vi "Wait for Win Msg.vi"(0 "win msg queue":T1, 1 "ms timeout (-1)":i32=-1, 2 "ignore previous (F)":bool, 3 "error in (no error)":errorcluster) -> (4 "Messages Remaining in Queue":i32, 5 "Sent":bool, 6 "win msg queue out":T1, 7 "Message":T2 {"Msg" format="%.0x"; "hWnd" format="%.0x"}, 8 "timed out":bool, 9 "error out":errorcluster)   [LabVIEW 2011]
doc: "Asynchronously waits for the next windows message that is added to the queue and returns it. If ignore previous is set to true, all messages occurring before this wait are deleted. If it is set to false and prior messages are waiting in the queue, this VI returns immediately with the next message. No more than one Wait per queue should be active at any given time. Simultaneous waits on different queues are permissible.\n\nParameters:\nwin msq queue: the queue for which to wait.\n\nms timeout: timeout time in milliseconds\n\niqnore previous: whether to pay attention to messages added to the queue before this VI begins waiting. If true, only the message added to the queue while the VI is waiting are detected. All other prior messages are deleted. If false, if one or more messages are posted before the VI begins waiting, this VI returns immediately with the oldest message in the queue.\n\ntimed out: returns true if the timeout expired.\n\nMessage: the oldest message in the queue is removed and returned. (Usually this is the only message in the queue.) See Get Next Message.vi for more information.\n\nSent: returns true if the returned message was sent to the window (via SendMessage) or false if it was posted (via PostMessage). Note: messages that are sent will not have valid time or point parameters.\n\nMessage Remaining: the number of messsages still in the queue.\n\nErrors:\n6751: not a valid windows message queue.\n6752: no messages in queue when read was attempted."
uses:
  Win Msg Q RefNum.ctl
  Win Msg.ctl
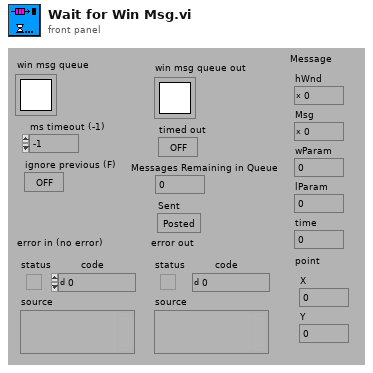
[diagram p1: front panel]
types:
  T1 = typedef "Win Msg Q RefNum.ctl" = refnum<k1>
  T2 = typedef "Win Msg.ctl" = cluster{"hWnd":u32, "Msg":u32, "wParam":u32, "lParam":i32, "time":u32, "point":cluster{"X":i32, "Y":i32}}
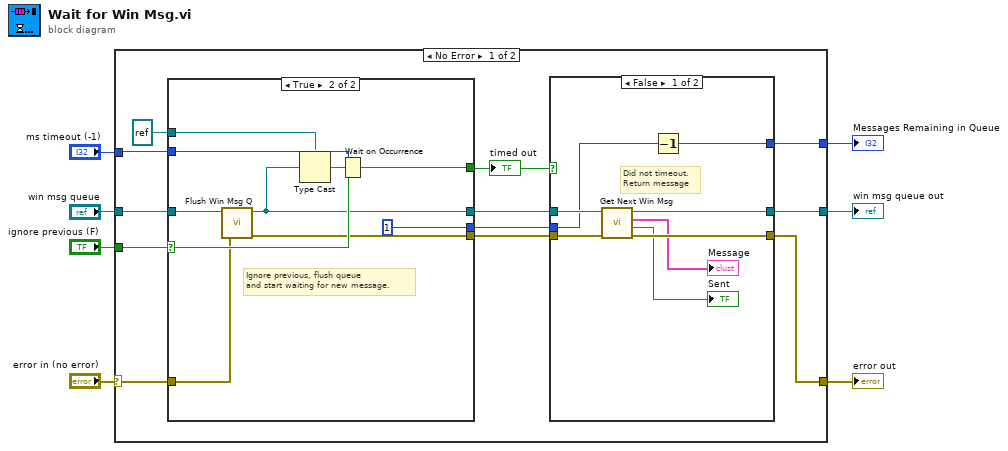
[diagram p0: block diagram]
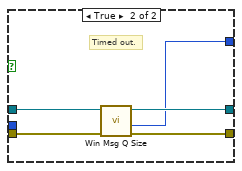
[diagram p2: hidden frame]
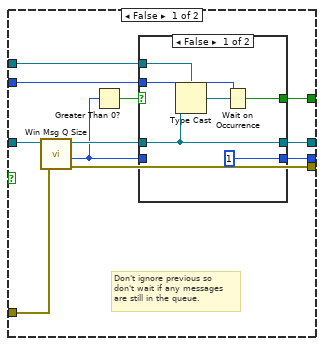
[diagram p3: hidden frame]
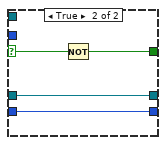
[diagram p4: hidden frame]
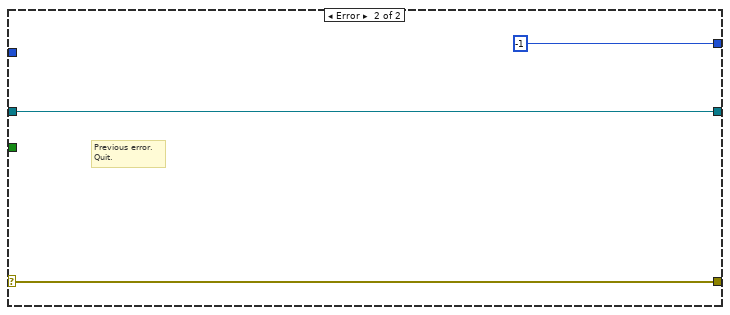
[diagram p5: hidden frame]
diagram:
  n1 = case shown="No Error" "error in (no error)" {
    selector: "error in (no error)" -> [w10 w64]
    tunnel: "win msg queue" -> [w18 w66]
    tunnel: "ms timeout (-1)" -> [w19 _]
    tunnel: "ignore previous (F)" -> [w17 _]
    tunnel: [w14 w66] -> w4
    tunnel: [w13 w64] -> w2
    tunnel: [w12 -1 ("Items in queue")] -> w3
    frame No Error {
      n2 = case shown="True" w17 {
        selector: w17 -> [_ w62]
        tunnel: w19 -> [w40 w61]
        tunnel: w18 -> [w43 w59]
        tunnel: [w39 w60] -> w9
        tunnel: [w38 w58] -> w16
        tunnel: [w37 w57] -> w15
        tunnel: [w35 1 ("Items in queue")] -> w11
        tunnel: w10 -> [w34 w55]
        tunnel: refnum<k4> refnum ("Occurrence RefNum") -> [w33 w54]
        frame False {
          # "Don't ignore previous so\ndon't wait if any messages\nare still in the queue."
          n3 = call "Win Msg Q Size.vi"("error in (no error)"=w34, "win msg queue"=w43) -> ("error out"=w37:errorcluster, "Items in queue"=w36:i32, "win msg queue out"=w41:T1)  [unwired: 3 out]
          n4 = Greater Than 0?(x=w36) -> (x > 0?=w42:bool)
          n5 = case shown="False" w42 {
            selector: w42 -> [_ w53]
            tunnel: [w49 w51] -> w39
            tunnel: w41 -> [w46 w52]
            tunnel: w40 -> [w47 _]
            tunnel: [w46 w52] -> w38
            tunnel: w36 -> [_ w50]
            tunnel: [1 ("Items in queue") w50] -> w35
            tunnel: w33 -> [w44 _]
            frame False {
              n6 = Type Cast(type=w44, x=w46) -> (*(type *) &x=w48:refnum<k4>)
              n7 = Wait on Occurrence(2:w48, 3:w47) -> (0:w49:bool)  [unwired: 1 out]
            }
            frame True {
              n8 = Not(x=w53) -> (.not. x?=w51:bool)
            }
          }
        }
        frame True {
          # "Ignore previous, flush queue\nand start waiting for new message."
          n9 = call "Flush Win Msg Q.vi"("error in (no error)"=w55, "win msg queue"=w59) -> ("error out"=w57:errorcluster, "win msg queue out"=w58:T1)  [unwired: 4 out]
          n10 = Type Cast(type=w54, x=w58) -> (*(type *) &x=w63:refnum<k4>)
          n11 = Wait on Occurrence(1:w62, 2:w63, 3:w61) -> (0:w60:bool)
        }
      }
      "timed out" <- w9
      n12 = case shown="False" w9 {
        tunnel: w16 -> [w27 w31]
        tunnel: w15 -> [w26 w32]
        tunnel: [w25 w30] -> w14
        tunnel: [w24 w29] -> w13
        tunnel: [w22 w28] -> w12
        tunnel: w11 -> [w23 _]
        frame False {
          # "Did not timeout.\nReturn message"
          n13 = call "Get Next Win Msg.vi"("error in (no error)"=w26, "win msg queue"=w27) -> ("error out"=w24:errorcluster, "Sent"=→"Sent":bool, "Message"=→"Message":T2, "win msg queue out"=w25:T1)  [unwired: 2 out]
          n14 = Decrement(x=w23) -> (x-1=w22:i32)
        }
        frame True {
          # "Timed out."
          n15 = call "Win Msg Q Size.vi"("error in (no error)"=w32, "win msg queue"=w31) -> ("error out"=w29:errorcluster, "Items in queue"=w28:i32, "win msg queue out"=w30:T1)  [unwired: 3 out]
        }
      }
    }
    frame Error {
      # "Previous error.\nQuit."
    }
  }
  "error out" <- w2
  "Messages Remaining in Queue" <- w3
  "win msg queue out" <- w4
